vi "Ctor.vi"(7 "Debug (F)":bool, 8 "error in (no error)":errorcluster, 9 "SSL Key Password (None)":string, 10 "HTTPS Options (Disabled)":T1={"HTTPS Enabled"=FALSE, "Private Key"=path "", "Private Key Format"=enum."PKCS#8 (PEM)", "Public Cert"=path "", "Public Cert Format"=enum."X.509 (PEM)", "Always Secure?"=TRUE, "HTTPS Port (443)"=433}, 11 "HTTP Port (80)":u16=80) -> (0 "error out":errorcluster, 3 "Server out":refnum<class "Server.lvclass">)   [LabVIEW 2020, in "HTTP Server.lvlib" / "Server.lvclass"]
uses:
  Server.lvclass
  Server.lvclass/Server.ctl
  Ref Data.ctl
  Exception Handler/Exception Handler.lvclass
  Priority.ctl
  HTTP Server.lvlib
  Exception Handler Map.ctl
  Complete Handler/Complete Handler.lvclass
  Complete Handler Map.ctl
  Response Handler/Response Handler.lvclass
  Response Handler Map.ctl
  Controller/Controller.lvclass
  Controller Map.ctl
  Controller Handler/Controller Handler.lvclass
  Controller Handler Map.ctl
  Route Handler/Route Handler.lvclass
  Route Handler Map.ctl
  Request Handler/Request Handler.lvclass
  Request Handler Map.ctl
  Connection Handler/Connection Handler.lvclass
  Connection Handler Map.ctl
  RequestTraceLog/RequestTraceLog.lvclass
  Values/Values.lvclass
  Session/Session.lvclass
  WebSocket Handler/WebSocket Handler.lvclass
  WebSocket Data.ctl
  lv-stream-websocket/Stream-Websocket/Websocket Server/Websocket Server.lvclass
  SSE Manager/SSE Manager.lvclass
  Server Sent Events Data.ctl
  lv-uri/URI/URI/URI.lvclass
  C:/dev/lv20CE/relink/lv-http-server/HTTP Server/Connection Handler/Connection Handler.lvclass
  C:/dev/lv20CE/relink/lv-http-server/HTTP Server/Handler/Handler.lvclass
  C:/dev/lv20CE/relink/lv-http-server/HTTP Server/Request Handler/Request Handler.lvclass
  C:/dev/lv20CE/relink/lv-http-server/HTTP Server/Route Handler/Route Handler.lvclass
  C:/dev/lv20CE/relink/lv-http-server/HTTP Server/Controller Handler/Controller Handler.lvclass
  C:/dev/lv20CE/relink/lv-http-server/HTTP Server/Controller/Controller.lvclass
  C:/dev/lv20CE/relink/lv-http-server/HTTP Server/Response Handler/Response Handler.lvclass
  C:/dev/lv20CE/relink/lv-http-server/HTTP Server/Complete Handler/Complete Handler.lvclass
  C:/dev/lv20CE/relink/lv-http-server/HTTP Server/Exception Handler/Exception Handler.lvclass
  C:/dev/lv20CE/relink/lv-http-server/HTTP Server/WebSocket Handler/WebSocket Handler.lvclass
  HTTPS Options.ctl
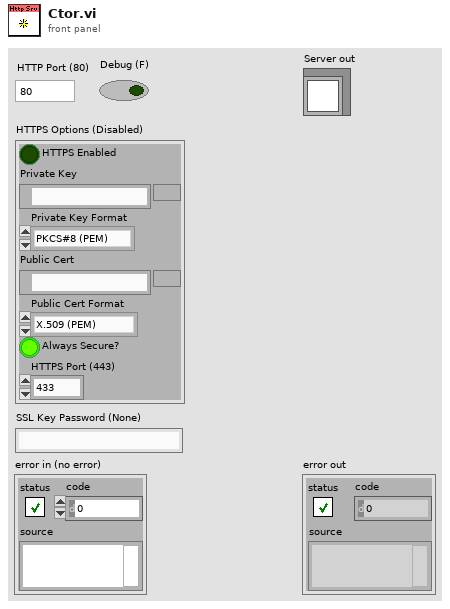
[diagram p1: front panel]
types:
  T1 = typedef "HTTP Server.lvlib/HTTPS Options.ctl" = cluster{"HTTPS Enabled":bool, "Private Key":path, "Private Key Format":enum32{"PKCS#8 (PEM)", "PKCS#8 (DER)"}, "Public Cert":path, "Public Cert Format":enum32{"X.509 (PEM)"}, "Always Secure?":bool, "HTTPS Port (443)":u16}
  T2 = typedef "HTTP Server.lvlib/Server Sent Events Data.ctl" = cluster{"Resources":map{string, refnum<class "SSE Manager.lvclass">}}
  T3 = typedef "HTTP Server.lvlib/WebSocket Data.ctl" = cluster{"Buffered WS Map":map{string, refnum<class "Websocket Server.lvclass">}, "Message WS Map":map{string, refnum<class "Websocket Server.lvclass">}}
  T4 = typedef "HTTP Server.lvlib/Server.lvclass/Ref Data.ctl" = cluster{"Connection Handler Map":T5, "Request Handler Map":T7, "Route Handler Map":T8, "Controller Handler Map":T9, "Controller Map":T10, "Response Handler Map":T11, "Complete Handler Map":T12, "Exception Handler Map":T13, "Connection Handler Index":u16, "Request Handler Index":u16, "Route Handler Index":u16, "Controller Handler Index":u16, "Controller Index":u16, "Response Handler Index":u16, "Complete Handler Index":u16, "Exception Handler Index":u16, "Values":refnum<class "Values.lvclass">, "Path":path, "Session Type":refnum<class "Session.lvclass">, "Session Cookie Name":string, "WebSocket Handler":refnum<class "WebSocket Handler.lvclass">, "WebSocket Handling":bool}
  T5 = typedef "HTTP Server.lvlib/Connection Handler Map.ctl" = map{T6, refnum<class "Connection Handler.lvclass">}
  T6 = typedef "HTTP Server.lvlib/Priority.ctl" = cluster{"Entity":u16, "Index":u16}
  T7 = typedef "HTTP Server.lvlib/Request Handler Map.ctl" = map{T6, refnum<class "Request Handler.lvclass">}
  T8 = typedef "HTTP Server.lvlib/Route Handler Map.ctl" = map{T6, refnum<class "Route Handler.lvclass">}
  T9 = typedef "HTTP Server.lvlib/Controller Handler Map.ctl" = map{T6, refnum<class "Controller Handler.lvclass">}
  T10 = typedef "HTTP Server.lvlib/Controller Map.ctl" = map{T6, refnum<class "Controller.lvclass">}
  T11 = typedef "HTTP Server.lvlib/Response Handler Map.ctl" = map{T6, refnum<class "Response Handler.lvclass">}
  T12 = typedef "HTTP Server.lvlib/Complete Handler Map.ctl" = map{T6, refnum<class "Complete Handler.lvclass">}
  T13 = typedef "HTTP Server.lvlib/Exception Handler Map.ctl" = map{T6, refnum<class "Exception Handler.lvclass">}
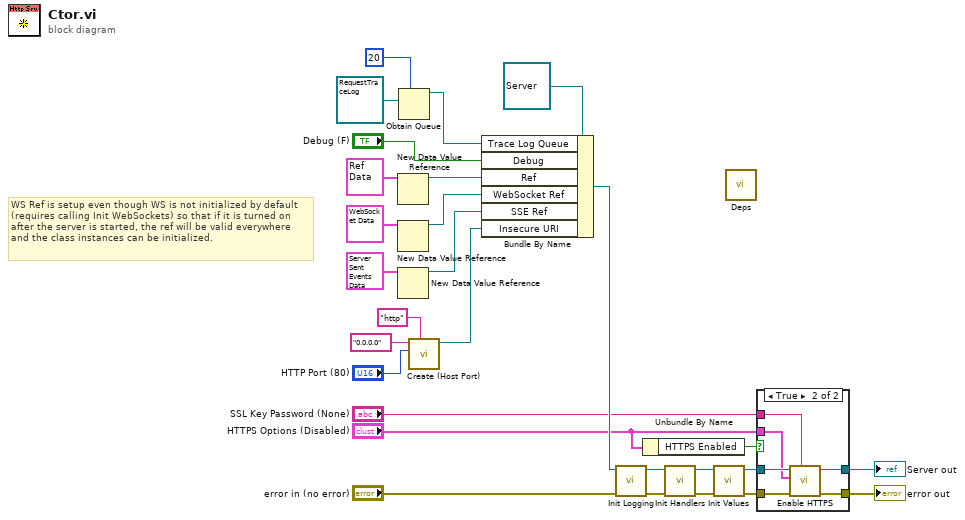
[diagram p0: block diagram]
diagram:
  # "WS Ref is setup even though WS is not initialized by default (requires calling Init WebSockets) so that if it is turned on after the server is started, the ref will be valid everywhere and the class instances can be initialized."
  n1 = New Data Value Reference(data value=T4 {"Connection Handler Map"={}, "Request Handler Map"={}, "Route Handler Map"={}, "Controller Handler Map"={}, "Controller Map"={}, "Response Handler Map"={}, "Complete Handler Map"={}, "Exception Handler Map"={}, "Connection Handler Index"=0, "Request Handler Index"=0, "Route Handler Index"=0, "Controller Handler Index"=0, "Controller Index"=0, "Response Handler Index"=0, "Complete Handler Index"=0, "Exception Handler Index"=0, "Values"=refnum, "Path"=path "", "Session Type"=refnum, "Session Cookie Name"="", "WebSocket Handler"=refnum, "WebSocket Handling"=FALSE} ("Ref Data")) -> (data value reference=w24:refnum<data-value>)  [unwired: 1 in, 1 out]
  n2 = New Data Value Reference(data value=T3 {"Buffered WS Map"={}, "Message WS Map"={}} ("WebSocket Data")) -> (data value reference=w16:refnum<data-value>)  [unwired: 1 in, 1 out]
  n3 = New Data Value Reference(data value=T2 {"Resources"={}} ("Server Sent Events Data")) -> (data value reference=w5:refnum<data-value>)  [unwired: 1 in, 1 out]
  n4 = Obtain Queue(max queue size (-1, unlimited)=20, element data type=refnum<class "RequestTraceLog.lvclass"> refnum ("HTTP Server.lvlib:RequestTraceLog.lvclass")) -> (queue out=w20:refnum<queue>)  [unwired: 3 in, 2 out]
  n5 = call "Create (Host Port).vi"("Scheme (None)"="http", "Port"="HTTP Port (80)", "Host"="0.0.0.0") -> ("URI out"=w3:refnum<class "URI.lvclass">)  [unwired: 8 in]
  n6 = Bundle By Name(cluster=refnum<class "Server.lvclass"> refnum ("Server in"), "Trace Log Queue"=w20, "Debug"="Debug (F)", "Ref"=w24, "WebSocket Ref"=w16, "SSE Ref"=w5, "Insecure URI"=w3) -> (w25:refnum<class "Server.lvclass">)
  n7 = call "Init Logging.vi"("error in (no error)"="error in (no error)", "Server in"=w25) -> ("error out"=w12:errorcluster, "Server out"=w13:refnum<class "Server.lvclass">)  [unwired: 8 in]
  n8 = Unbundle By Name("HTTPS Options (Disabled)") -> ("HTTPS Enabled"=w7:bool)
  n9 = call "Init Handlers.vi"("error in (no error)"=w12, "Server in"=w13) -> ("error out"=w18:errorcluster, "Server out"=w19:refnum<class "Server.lvclass">)  [unwired: 8 in]
  n10 = call "Init Values.vi"("error in (no error)"=w18, "Server in"=w19) -> ("error out"=w10:errorcluster, "Server out"=w11:refnum<class "Server.lvclass">)  [unwired: 8 in]
  n11 = call "Deps.vi"() -> ()  [unwired: 12 in]
  n12 = case shown="True" w7 {
    tunnel: w11 -> [w30 w36]
    tunnel: w10 -> [w29 w35]
    tunnel: "SSL Key Password (None)" -> [_ w34]
    tunnel: [w30 w33] -> w15
    tunnel: [w29 w32] -> w14
    tunnel: "HTTPS Options (Disabled)" -> [_ w31]
    frame False {
    }
    frame True {
      n13 = call "Enable HTTPS.vi"("Private Key Password (None)"=w34, "error in (no error)"=w35, "HTTPS Options"=w31, "Server in"=w36) -> ("error out"=w32:errorcluster, "Server out"=w33:refnum<class "Server.lvclass">)  [unwired: 6 in]
    }
  }
  "error out" <- w14
  "Server out" <- w15
